vi "2-input X-OR.vi"(10 "Obtained Expression":string, 11 "Input List":string[](array[string])) -> (2 "X-OR ?":bool, 3 "Logic Exp":string)   [LabVIEW 2014]
doc: "This VI is used to compare the obtained logic with the logic of NAND gate."
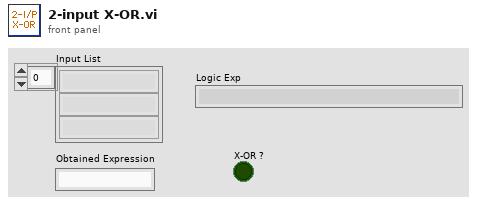
[diagram p1: front panel]
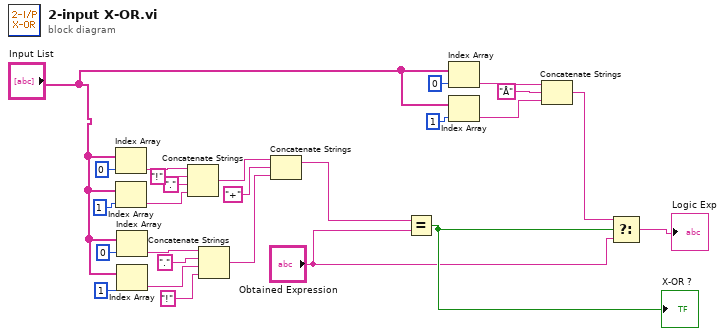
[diagram p0: block diagram]
diagram:
  n1 = Index Array(array="Input List", index=0) -> (element=w17:string)
  n2 = Index Array(array="Input List", index=1) -> (element=w14:string)
  n3 = Index Array(array="Input List", index=0) -> (element=w23:string)
  n4 = Index Array(array="Input List", index=1) -> (element=w25:string)
  n5 = Concatenate Strings(w17, "!" ("t"), "." ("string"), w14) -> (w19:string)
  n6 = Concatenate Strings(w23, "." ("string"), w25, "!" ("string")) -> (w26:string)
  n7 = Concatenate Strings(w19, "+" ("string"), w26) -> (w12:string)
  n8 = Equal?(x=w12, y="Obtained Expression") -> (x = y?=w11:bool)
  "X-OR ?" <- w11
  n9 = Index Array(array="Input List", index=0) -> (element=w7:string)
  n10 = Index Array(array="Input List", index=1) -> (element=w5:string)
  n11 = Concatenate Strings(w7, "Å" ("string"), w5) -> (w4:string)
  n12 = Select(t=w4, s=w11, f="Obtained Expression") -> (s? t:f=→"Logic Exp":string)
